vi "Calculate Power from Joystick Tank v2_Threashold.vi"(4 "lower limit":i32, 5 "upper limit":i32=100, 6 "Reverse":bool, 7 "Deadband (10)":i32=10 max=100 step=1, 8 "Throttle (50)":i32=50 min=0 max=100 step=1, 9 "Right Joystick":i32, 10 "Left Joystick":i32, 11 "NXT":T1) -> (0 "Power 2":i8, 2 "Power 1":i8, 3 "NXT":T1)   [LabVIEW 2012]
doc: "Determines the amount of power to apply to a pair of motors according to the y- values of each joystick on a controller. When calculating the amount of power to apply, this VI scales the joystick values to values a motor can accept.\n\nNote: This VI only performs math. It does not read from joystick hardware or write to motors.\n\nUse this VI to drive the robot with two joysticks on a controller. Select Arcade Steering from the polymorphic selector below the VI icon to drive the robot with one joystick.\n\n<B>Inputs</B>\n<B>Deadband</B> specifies the joystick values that the VI treats as 0. When the position of the joystick is within the range you specify, the VI considers the joystick to be at position 0. The default range is -10 to 10.\n<B>NXT</B> establishes the flow of the program. Wire the <B>NXT</B> output of the previous VI in the program to the <B>NXT</B> input of this VI.\n<B>Left Joystick</B> specifies the y-axis value of the left joystick on the controller. You can specify a value between -127 and 127.\n<B>Right Joystick</B> specifies the y-axis value of the right joystick on the controller. You can specify a value between -127 and 127.\n<B>Throttle</B> scales the range of power that can be applied to the motors. For example, a throttle value of 50 scales the full range of the joystick to 50 percent. You can specify a value of -100 to 100. A negative number switches the drive motors, meaning the back of the robot becomes the front of the robot. A value of 0 specifies that the motor does not move, and 100 specifies the fastest motor speed. The default is 50.\n<B>Reverse</B> specifies, when TRUE, that the motors move in the reverse direction. The default is FALSE.\n\n<B>Outputs</B>\n<B>NXT</B> establishes the flow of the program. Wire the <B>NXT</B> output of this VI to the <B>NXT</B> input of the next VI in the program.\n<B>Power 1</B> returns the power to apply to motor 1.\n<B>Power 2</B> returns the power to apply to motor 2."
uses:
  <vilib>/NXT/Subs/LVHSConnector.ctl
  <vilib>/NXT/LegoClasses/BrickReference/BrickReference.lvclass
  <vilib>/NXT/Dual Mode Library/prims/inRangeAndCoerce/inRangeAndCoerce_int.vi
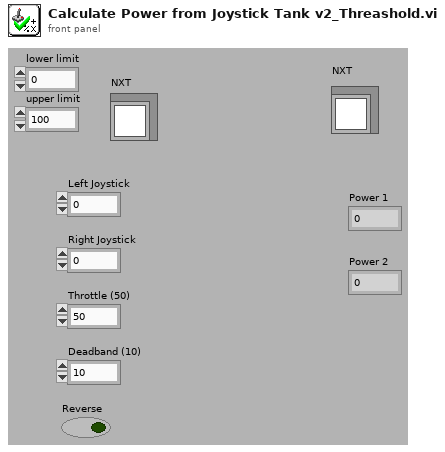
[diagram p1: front panel]
types:
  T1 = typedef "LVHSConnector.ctl" = refnum<class "BrickReference.lvclass">
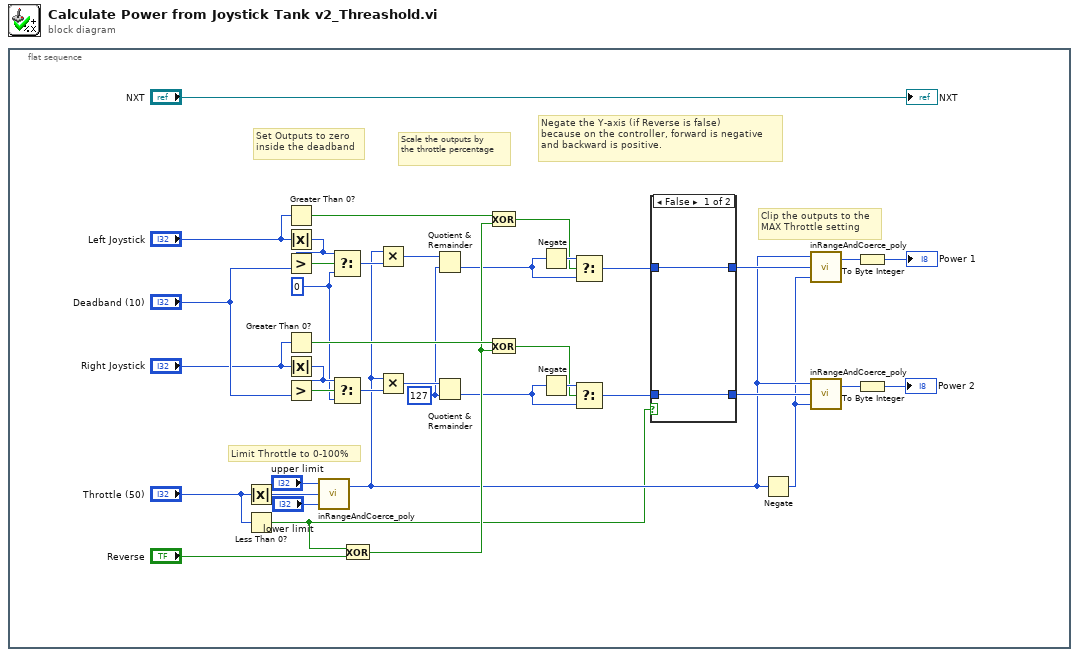
[diagram p0: block diagram]
diagram:
  n1 = flat-sequence {
    frame #0 {
      w12 = 127
      w13 = 0 ("f")
      # "Limit Throttle to 0-100%"
      # "Scale the outputs by\nthe throttle percentage"
      # "Clip the outputs to the\nMAX Throttle setting"
      # "Set Outputs to zero\ninside the deadband"
      # "Negate the Y-axis (if Reverse is false) \nbecause on the controller, forward is negative\nand backward is positive."
      n2 = Absolute Value(x="Throttle (50)") -> (abs(x)=w29:i32)
      n3 = Less Than 0?(x="Throttle (50)") -> (x < 0?=w16:bool)
      n4 = Greater Than 0?(x="Left Joystick") -> (x > 0?=w26:bool)
      n5 = Absolute Value(x="Left Joystick") -> (abs(x)=w15:i32)
      n6 = Greater?(x=w15, y="Deadband (10)") -> (0:w38:bool)
      n7 = Greater Than 0?(x="Right Joystick") -> (x > 0?=w27:bool)
      n8 = Absolute Value(x="Right Joystick") -> (abs(x)=w14:i32)
      n9 = Greater?(x=w14, y="Deadband (10)") -> (0:w33:bool)
      n10 = call-poly <vilib>:"inRangeAndCoerce_poly.vi"("lower limit"="lower limit", "x"=w29, "upper limit"="upper limit") -> ("coerced(x)"=w22:i32)  [unwired: 1 out]
      n11 = Select(t=w15, s=w38, f=w13) -> (s? t:f=w37:i32)
      n12 = Select(t=w14, s=w33, f=w13) -> (s? t:f=w34:i32)
      n13 = Exclusive Or(1:"Reverse", 2:w16) -> (0:w25:bool)
      n14 = Multiply(x=w22, y=w37) -> (x*y=w36:i32)
      n15 = Multiply(x=w22, y=w34) -> (x*y=w35:i32)
      n16 = Quotient & Remainder(x=w36, y=w12) -> (floor(x/y)=w6:i32)  [unwired: 1 out]
      n17 = Quotient & Remainder(x=w35, y=w12) -> (floor(x/y)=w2:i32)  [unwired: 1 out]
      n18 = Exclusive Or(1:w25, 2:w26) -> (0:w5:bool)
      n19 = Exclusive Or(1:w25, 2:w27) -> (0:w1:bool)
      n20 = Negate(x=w6) -> (-x=w7:i32)
      n21 = Negate(x=w2) -> (-x=w4:i32)
      n22 = Select(t=w7, s=w5, f=w6) -> (s? t:f=w8:i32)
      n23 = Select(t=w4, s=w1, f=w2) -> (s? t:f=w3:i32)
      n24 = case shown="False" w16 {
        tunnel: w8 -> [w41 w42]
        tunnel: [w41 w43] -> w24
        tunnel: [w40 w42] -> w23
        tunnel: w3 -> [w40 w43]
        frame False {
        }
        frame True {
        }
      }
      n25 = Negate(x=w22) -> (-x=w21:i32)
      n26 = call-poly <vilib>:"inRangeAndCoerce_poly.vi"("lower limit"=w21, "x"=w24, "upper limit"=w22) -> ("coerced(x)"=w20:i32)  [unwired: 1 out]
      n27 = call-poly <vilib>:"inRangeAndCoerce_poly.vi"("lower limit"=w21, "x"=w23, "upper limit"=w22) -> ("coerced(x)"=w19:i32)  [unwired: 1 out]
      n28 = To Byte Integer(number=w20) -> (8bit integer=→"Power 1":i8)
      n29 = To Byte Integer(number=w19) -> (8bit integer=→"Power 2":i8)
      "NXT" <- "NXT"
    }
  }
